vi "Untitled 20(SubVI).vi"(4 "Numeric 2":dbl, 6 "Numeric out 3":dbl, 7 "Numeric in":dbl, 9 "Numeric":dbl, 10 "Numeric in":dbl, 11 "Numeric 4":dbl) -> (2 "Numeric 3":dbl, 3 "Numeric 5":dbl)   [LabVIEW 2019]
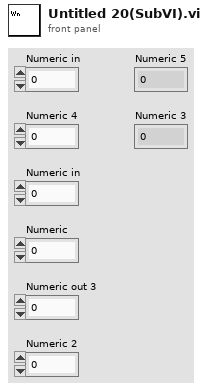
[diagram p1: front panel]
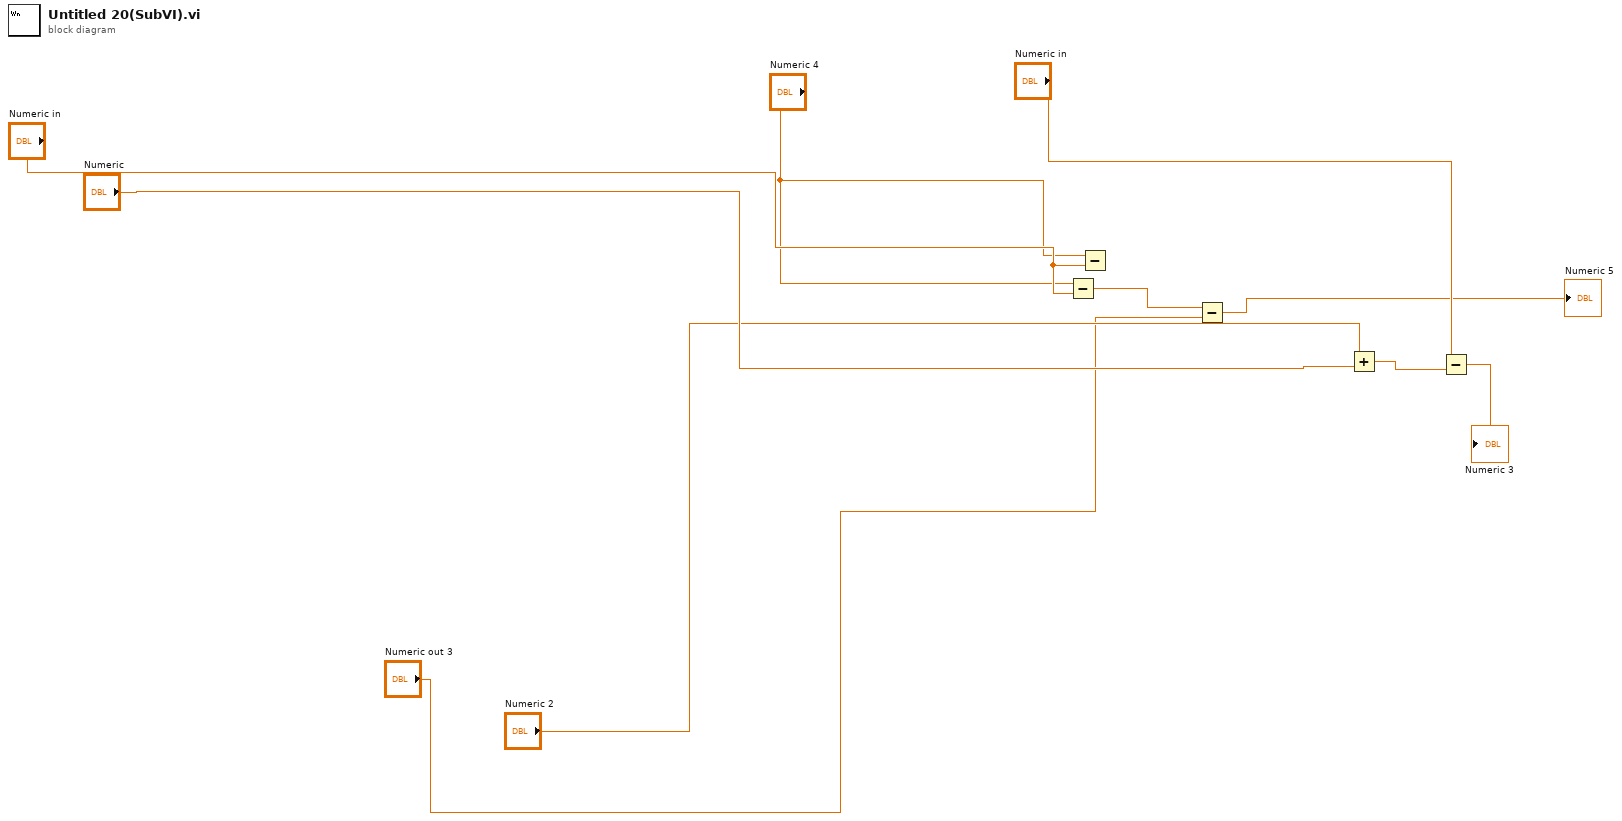
[diagram p0: block diagram]
diagram:
  n1 = Subtract(x="Numeric 4", y="Numeric in") -> (x-y=w1:dbl)
  n2 = Subtract(x="Numeric 4", y="Numeric in") -> ()  [unwired: 1 out]
  n3 = Subtract(x=w1, y="Numeric out 3") -> (x-y=→"Numeric 5":dbl)
  n4 = Add(x="Numeric 2", y="Numeric") -> (x+y=w9:dbl)
  n5 = Subtract(x="Numeric in", y=w9) -> (x-y=→"Numeric 3":dbl)
